vi "MB Ethernet Slave Demon - Single Port - Multiple Connections 2.vi"(9 "Period":u32=75, 10 "Timeout":i32=5000, 11 "Port":u16=502) -> (2 "Demon Running":bool, 3 "# of connections":i32)   [LabVIEW 2023, in "Voegtlin_NI_SMART_Modbus_Drivers.lvlib"]
uses:
  Voegtlin_NI_SMART_Modbus_Drivers.lvlib
  MB RefCount Function.ctl
  MB Ethernet Connection Function.ctl
  <vilib>/Platform/TimedLoop/XDataNode/timing_clust.ctl
  <vilib>/Platform/TimedLoop/XDataNode/nitl_modes.ctl
  <vilib>/Platform/TimedLoop/XDataNode/wakeup.ctl
  MB Globals.vi
  <vilib>/Platform/TimedLoop/XDataNode/XDataNode.xnode
  <vilib>/Platform/TimedLoop/XDataNode/XDNodeRunTimeDep.lvlib
panel:
  in  "Case Constant\n(See Context Help)":bool
  # "VI Name: MB Ethernet Slave Demon.vi\nPurpose: Modbus Demon\nMonitor a single port, but can accept multiple connections."
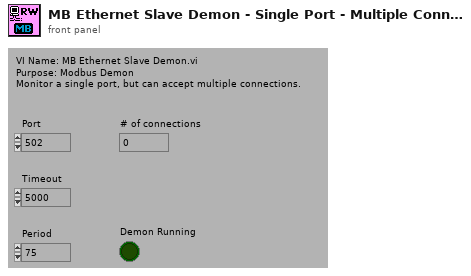
[diagram p1: front panel]
types:
  T1 = typedef "Voegtlin_NI_SMART_Modbus_Drivers.lvlib/MB RefCount Function.ctl" = enum16{"Init", "Add", "Remove", "Is Running?"}
  T2 = typedef "Voegtlin_NI_SMART_Modbus_Drivers.lvlib/MB Ethernet Connection Function.ctl" = enum16{"Init", "Add Connection", "Get All Connections", "Delete Connection"}
  T3 = typedef "XDNodeRunTimeDep.lvlib/timing_clust.ctl" = cluster{"Expected End [f-1]":u64, "Actual End [f-1]":u64, "Finished Late? [f-1]":bool, "Expected End [i-1]":u64, "Actual End [i-1]":u64, "Finished Late? [i-1]":bool, "Expected Start [i]":u64, "Actual Start [i]":u64, "Expected Start [f]":u64, "Actual Start [f]":u64, "Source Name":string, "Structure Name":string, "Period":i64, "Deadline":i64, "Offset":i64, "Start":i64, "Priority":i32, "Timeout":i32, "Mode":T4, "Wakeup Reason":T5, "Error":errorcluster, "Source Type":string, "Secondary Source Type":string, "Global End Time":u64, "Global Start Time":u64, "Frame Duration":u64, "Iteration Duration":u64, "Assigned CPU":i32, "I/O Scan Engine Mode":u32}
  T4 = typedef "XDNodeRunTimeDep.lvlib/nitl_modes.ctl" = enum32{"No Change", "Process missed periods, maintain original phase", "Discard missed periods, maintain original phase", "Process missed periods, ignore original phase", "Discard missed periods, ignore original phase"}
  T5 = typedef "XDNodeRunTimeDep.lvlib/wakeup.ctl" = enum32{"Normal", "Aborted", "Asynchronous wakeup", "Timing source error", "Timed loop error", "Timeout"}
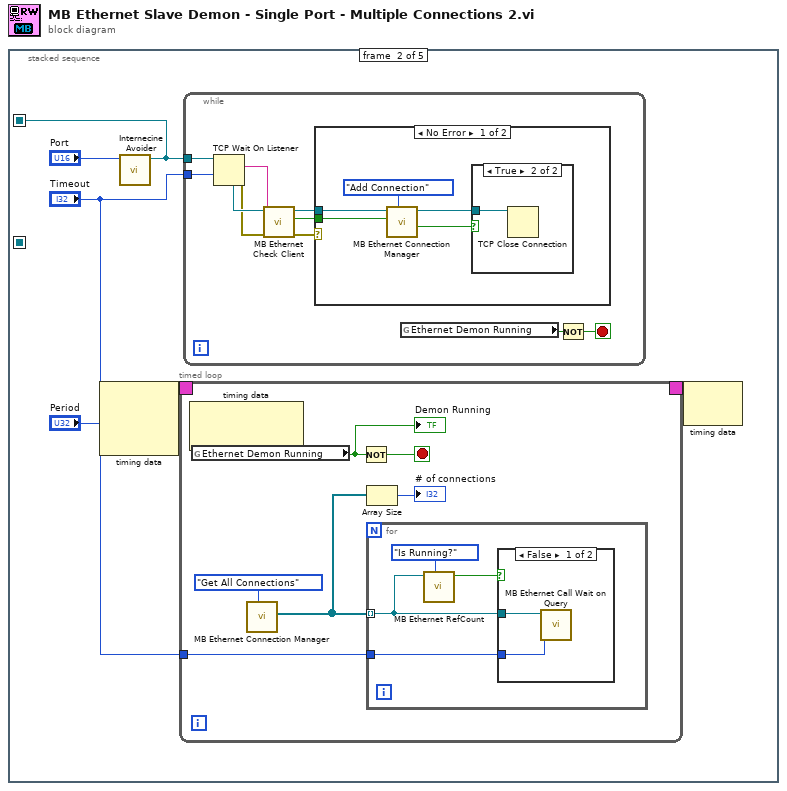
[diagram p0: block diagram]
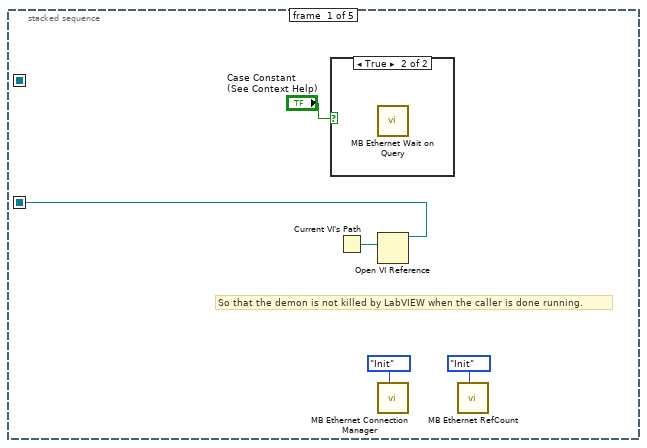
[diagram p2: hidden frame]
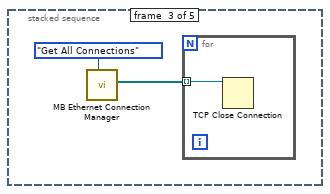
[diagram p7: hidden frame]
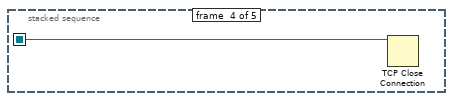
[diagram p8: hidden frame]
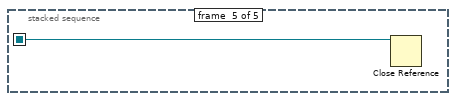
[diagram p9: hidden frame]
diagram:
  n1 = stacked-sequence {
    seq-local: [w4 _ _ _ _] -> [_ _ _ _ w50]
    seq-local: [_ w8 _ _ _] -> [_ _ _ w49 _]
    frame #0 {
      # "So that the demon is not killed by LabVIEW when the caller is done running."
      n2 = case shown="True" "Case Constant\n(See Context Help)" {
        frame False {
        }
        frame True {
          n3 = call "MB Ethernet Wait on Query.vi"() -> ()  [unwired: 2 in, 10 out]
        }
      }
      n4 = Current VI's Path() -> (path=w5:path)
      n5 = Open VI Reference(vi path=w5) -> (vi reference=w4:refnum<vi>)  [unwired: 1 in, 5 out]
      n6 = call "MB Ethernet Connection Manager.vi"("Function"=MB_Ethernet_Connection_Function."Init") -> ()  [unwired: 2 in, 9 out]
      n7 = call "MB Ethernet RefCount.vi"("Function"=MB_RefCount_Function."Init") -> ()  [unwired: 1 in, 10 out]
    }
    frame #1 {
      n8 = node-c288("Period") -> (w6:T3)  [unwired: 2 out]
      n9 = call <vilib>:"Internecine Avoider.vi"("port"="Port") -> ("connection ID"=w8:refnum<k5>)  [unwired: 3 in, 7 out]
      n10 = timed-loop {
        tunnel: "Timeout" -> [w12]
        timing-out: [_] -> w7
        timing: w6 -> [_]
        stop <- w17 stop-if-true
        n11 = node-c288() -> ()  [unwired: 3 out]
        n12 = global read "MB Globals.vi" "Ethernet Demon Running"() -> (w16:bool)
        "Demon Running" <- w16
        n13 = call "MB Ethernet Connection Manager.vi"("Function"=MB_Ethernet_Connection_Function."Get All Connections") -> ("Connection IDs"=w13:refnum<k5>[])  [unwired: 2 in, 8 out]
        n14 = Not(x=w16) -> (.not. x?=w17:bool)
        n15 = Array Size(array=w13) -> (size(s)=→"# of connections":i32)
        n16 = for {
          tunnel: w13 -> [w20] mode=indexing
          tunnel: w12 -> [w21]
          n17 = call "MB Ethernet RefCount.vi"("Function"=MB_RefCount_Function."Is Running?", "Connection ID"=w20) -> ("VI Running?"=w19:bool)  [unwired: 9 out]
          n18 = case shown="False" w19 {
            tunnel: w20 -> [w24 _]
            tunnel: w21 -> [w23 _]
            frame False {
              n19 = call "MB Ethernet Call Wait on Query.vi"("Timeout"=w23, "Connection ID"=w24) -> ()  [unwired: 10 out]
            }
            frame True {
            }
          }
        }
      }
      n20 = while {
        tunnel: w8 -> [w39]
        tunnel: "Timeout" -> [w36]
        stop <- w37 stop-if-true
        n21 = TCP Wait On Listener(9:w36, 11:w39) -> (0:w33:errorcluster, 2:w31:string, 4:w35:refnum<k5>)  [unwired: 1 in, 3 out]
        n22 = call "MB Ethernet Check Client.vi"("error in (no error)"=w33, "Remote Address"=w31, "Connection ID in"=w35) -> ("error out"=w32:errorcluster, "Priority"=w30:bool, "Connection ID out"=w34:refnum<k5>)  [unwired: 6 out]
        n23 = case shown="No Error" w32 {
          tunnel: w34 -> [w44 _]
          tunnel: w30 -> [w40 _]
          frame No Error {
            n24 = call "MB Ethernet Connection Manager.vi"("Function"=MB_Ethernet_Connection_Function."Add Connection", "Priority"=w40, "Connection ID"=w44) -> ("Close Connection"=w42:bool, "Connection ID to Delete"=w41:refnum<k5>)  [unwired: 7 out]
            n25 = case shown="True" w42 {
              tunnel: w41 -> [_ w45]
              frame False {
              }
              frame True {
                n26 = TCP Close Connection(connection ID=w45) -> ()  [unwired: 1 in, 3 out]
              }
            }
          }
          frame Error {
          }
        }
        n27 = global read "MB Globals.vi" "Ethernet Demon Running"() -> (w38:bool)
        n28 = Not(x=w38) -> (.not. x?=w37:bool)
      }
      n29 = node-c288(w7) -> ()  [unwired: 1 out]
    }
    frame #2 {
      n30 = call "MB Ethernet Connection Manager.vi"("Function"=MB_Ethernet_Connection_Function."Get All Connections") -> ("Connection IDs"=w46:refnum<k5>[])  [unwired: 2 in, 8 out]
      n31 = for {
        tunnel: w46 -> [w48] mode=indexing
        n32 = TCP Close Connection(connection ID=w48) -> ()  [unwired: 1 in, 3 out]
      }
    }
    frame #3 {
      n33 = TCP Close Connection(connection ID=w49) -> ()  [unwired: 1 in, 3 out]
    }
    frame #4 {
      n34 = Close Reference(reference=w50) -> ()  [unwired: 1 in, 1 out]
    }
  }
